vi "Gamma0.vi"(10 "Value":u32) -> (2 "Gamma 0":u32)   [LabVIEW 2018, in "Crypto.lvlib" / "SHA-256.lvclass"]
uses:
  SHA-256.lvclass
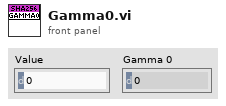
[diagram p1: front panel]
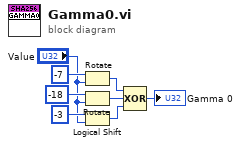
[diagram p0: block diagram]
diagram:
  n1 = Rotate(1:"Value", 2:i16 -7 ("y")) -> (0:w5:u32)
  n2 = Rotate(1:"Value", 2:i16 -18 ("y")) -> (0:w4:u32)
  n3 = Logical Shift(y=i16 -3, x="Value") -> (x << y=w2:u32)
  n4 = Compound Arithmetic op=XOR(w5, w4, w2) -> (→"Gamma 0":u32)
